vi "1D Scan.vi"(0 "System No.":i32=1 min=1 step=1, 1 "Analog In No.":i32=1 min=1 max=5 step=1, 2 "Axis to scan":string="Y", 4 "posdig":i16=4 caption="Digits" min=0 max=10 step=1, 5 "Scan direction":u16(ring) items=["Scan left & right (- & +)", "Scan only left (-)", "Scan only right (+)"], 6 "StartScan":bool, 7 "error in":errorcluster, 8 "Range":dbl=0.02 format="%.6f", 9 "Step size":dbl=0.002 format="%.6f", 12 "#6 polling?":bool=TRUE, 13 "Use MWG?":bool, 14 "VMO check?":bool=TRUE, 15 "Exit":bool, 16 "#5 Polling, ms":u32=10, 17 "Goto max":bool, 18 "Stop refnum":refnum<vi>) -> (20 "1D Array I":dbl[](array[numeric])=[0.00122, 0.00107, 0.00122, 0.00122, 0.56916, 1.88952, 3.75631, 5.80362, 5.80926, 3.7557, 1.89136, 0.56703, 0.00305, 0.00137, 0.00183] format="%.6f", 21 "1D Array X":dbl[](array[numeric])=[0.384, 0.386, 0.388, 0.39, 0.392, 0.394, 0.396, 0.398, 0.4, 0.402, 0.404, 0.406, 0.40800000000000003, 0.41000000000000003, 0.41200000000000003] format="%.6f", 23 "Intensity":cluster{dbl, dbl}(slide) scale=-1.0..0.00926 scale format="%.1f", 24 "Position":dbl format="%.6f", 27 "error out":errorcluster)   [LabVIEW 2011]
doc: "This VI performs a one-dimensional (1D) scan along one axis while monitoring an analog signal. The direction of the scan can be selected. After the scan, the axis to scan is optionally moved to the start position or to the position where the maximum occurred. The range and step size can be specified. After the scan, the axis can be moved to the maximum intensity position. Run XXX_Configuration_Setup.vi before starting this VI. \n\nStart the VI and select the system number (System No. = 1 in a one-system configuration) and Analog In number (Analog In No. = number of the analog channel to observe). Pressing Select will open a user interface which shows a list box with all axes connected to the selected system. Choose the axis to scan here or type the ID of the axis to scan directly into the Axis to scan control. Then, select Range and Step size for the scan. Digits is the number of digits after the decimal point in the position values that will be sent. #5 Polling is the cycle time in ms of the polling used to determine if motion has stopped after commanding a move. If this value is too large, scans may last very long. Set Scan orientation as needed (see possible orientations below). If #6 polling is on, VI will poll for position changes when idle. See control descriptions below to determine whether your system supports #6 polling. If MWG is on, the VI will use \"MWG.vi\" instead of \"MOV.vi\". This will result in a faster scan for systems which support the MWG command. See control descriptions below to determine if your system supports MWG. If VMO check is on, the VI will check whether the minimum and maximum position values of the scan line are within the system workspace before starting the scan. It is assumed that all positions between these points are reachable. See control descriptions below to determine whether your system supports VMO.\nIntensity graph shows the scanned intensity distribution. Autoscale can be switched on or off. If Autoscale is off, intensity is scaled from 0-10. \nPress Goto max to go to the position where the maximum intensity was found during the scan. With Clear max. the intensity value and the position value for the maximum intensity can be cleared. Press Save data to save scan data (axis, position and intensity information). Data will be saved in GCS Array format. With Save JPG a screen copy of this VI can be saved as a JPG file.\nPosition-Intensity Table will show the position value of the axis to scan and the corresponding intensity value which was captured during the scan. On the right side of the VI panel, the current and maximum intensity values and the current position value are shown.\nPress Stop to stop the scan and Exit to stop execution of this VI.\nTo use this VI as a sub-VI for your application without user interaction, wire the desired scan parameters (Axis to scan, Range, Step size, No. of pos. dig., #5 polling, #6 polling?, Use MWG?, VMO check?) to the corresponding terminals, and wire a TRUE constant to the Start scan, Goto max and Exit terminals. After calling the VI, it will make a scan, go to the maximum of the intensity distribution and finish execution. \n\nScan direction can be \n0: Left & right (- & +) meaning that the scan starts at \n(Start position - ½ Range) and stops at \n(Start position + ½ Range), \n1: To the left (-) meaning that scan starts at \n(Start position - Range) and stops at Start position, or \n2: To the right (+) meaning that scan starts at Start position and stops at (Start position + Range).\n\nWhen using as a sub-VI, connect Stop refnum terminal to stop VI from caller.\n\nValid for C-866, C-867, C-880, E-761, E-861, F-206, M-8X0, Mercury_GCS\n\nC-866: #6 polling? = FALSE, Use MWG? =FALSE, VMO check? =FALSE\nC-867: #6 polling? = FALSE, Use MWG? =FALSE, VMO check? =FALSE\nC-880: #6 polling? = TRUE, Use MWG? = FALSE, VMO check? = TRUE\nE-761: #6 polling? = TRUE, Use MWG? = FALSE, VMO check? = FALSE\nE-861: #6 polling? = FALSE, Use MWG? =FALSE, VMO check? =FALSE\nF-206: #6 polling? = TRUE, Use MWG? = TRUE, VMO check? = TRUE\nM-8X0: #6 polling? = TRUE, Use MWG? = FALSE, VMO check? = TRUE\nMercury_GCS: #6 polling? = FALSE, Use MWG? =FALSE, VMO check? = FALSE"
panel:
  in  "Save panel":bool
  in  "Autoscale":bool=TRUE
  out "No. of steps":i32=15
  out "Pos. Array":dbl[](array[numeric])=[0.398] caption="Start pos. array" format="%.6f"
  in  "Clear Max.":bool
  out "Start position":dbl=0.398 format="%.6f"
  out "Index of axis\nin Global 2":i32=1
  in  "Sub frame":i32=1
  in  "Select  axis":bool
  out "error":bool
  in  "StopAlign":bool
  in  "Next frame":i32
  in  "Save data":bool
  out "Position-Intensity Table":string[][](table)
  out "Intensity Graph":cluster{"1D Array X":dbl[], "1D Array Y":dbl[]}(graph) caption="No. of steps:"
  # "1D Scan"
  # "Run \"XXXX_Configuration_Setup.vi\" prior to running this VI. Scroll down for error clusters."
  # "Curr. I"
  # "Max. I"
  # "Error clusters and system specific settings"
  # "VI internal controls (do not change):"
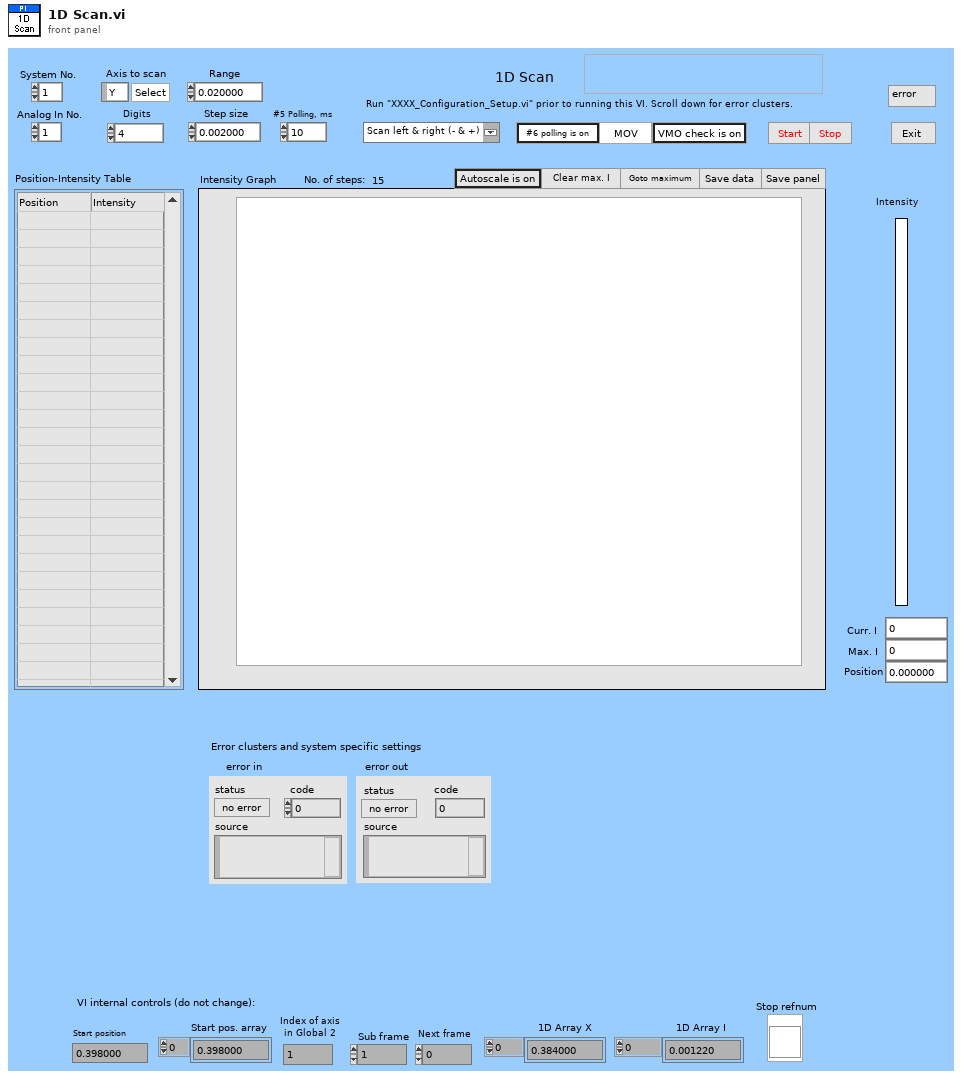
[diagram p1: front panel]
types:
  T1 = cluster{"Minimum":dbl, "Maximum":dbl, "Increment":dbl}
  T2 = cluster{"XName":string, "YName":string, "ZName":string}
  T3 = cluster{"Separator":string, "Remarks":string, "NDim":i32}
  T4 = cluster{"Read (F)/ Write":bool, "Path":path, "Datastream":string, "ArrayName":string}
  T5 = typedef "LVRectTypeDef.ctl" = cluster{"left":i16, "top":i16, "right":i16, "bottom":i16}
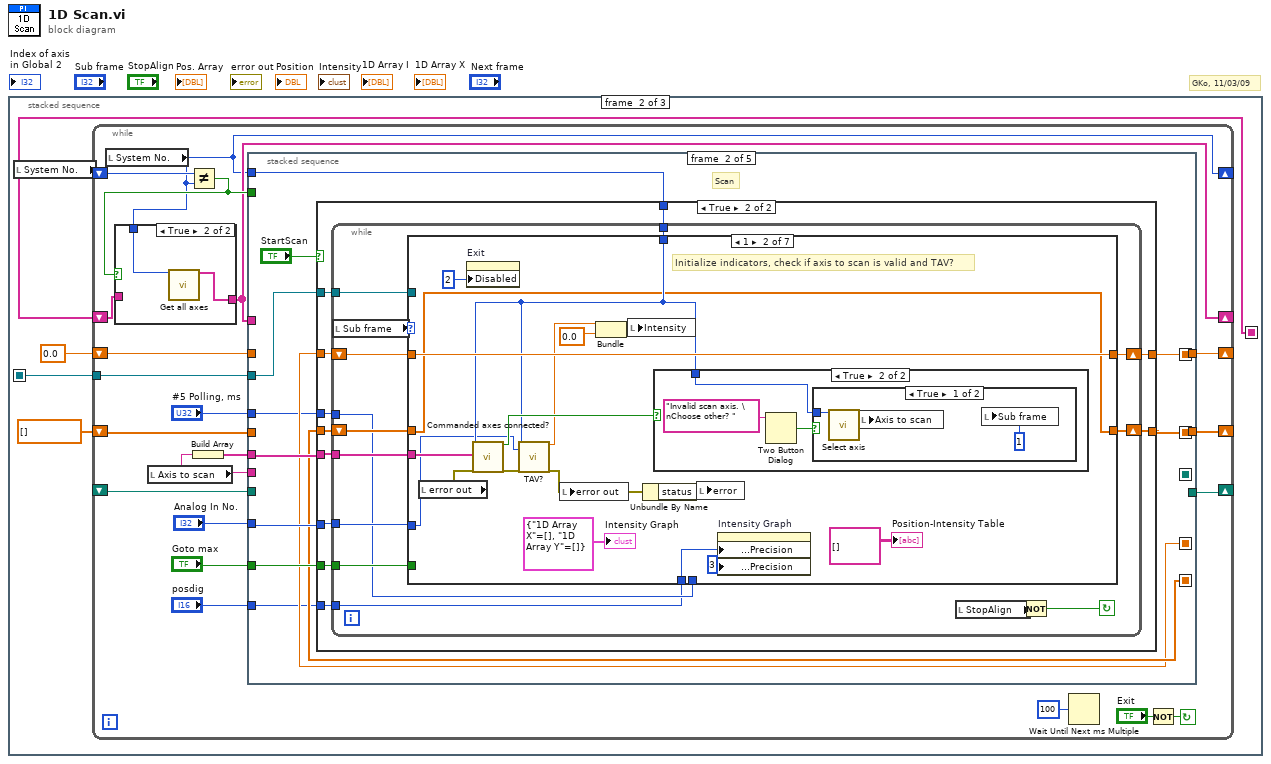
[diagram p0: block diagram]
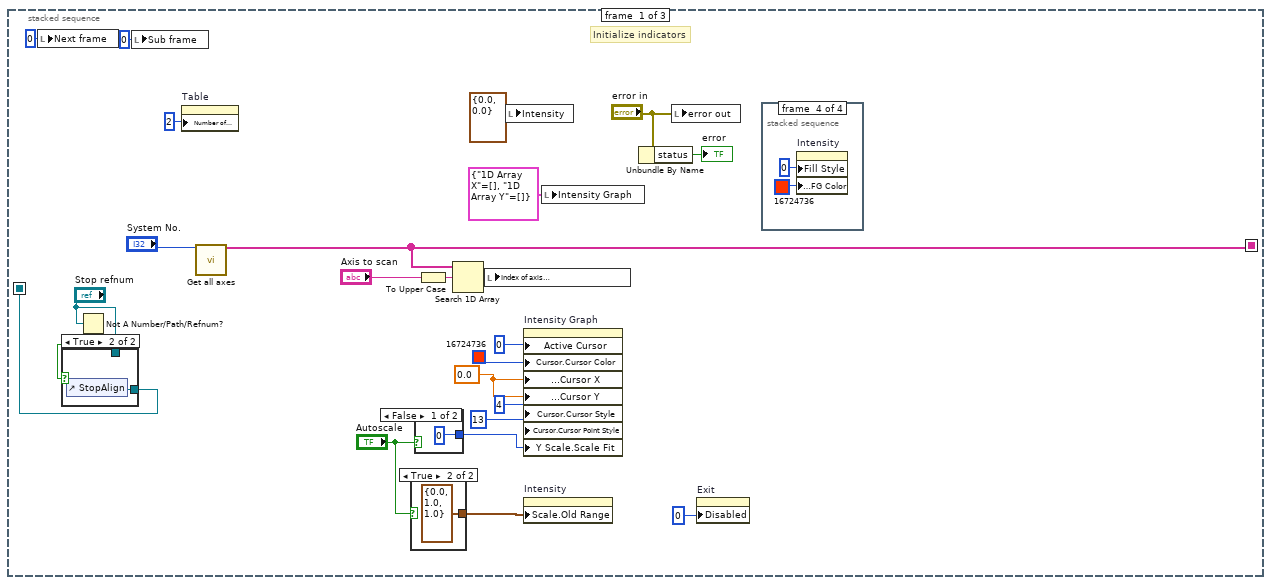
[diagram p2: hidden frame]
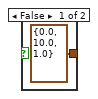
[diagram p3: hidden frame]
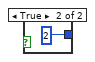
[diagram p5: hidden frame]
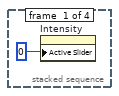
[diagram p6: hidden frame]
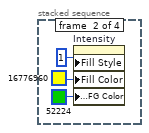
[diagram p7: hidden frame]
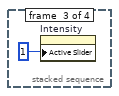
[diagram p8: hidden frame]
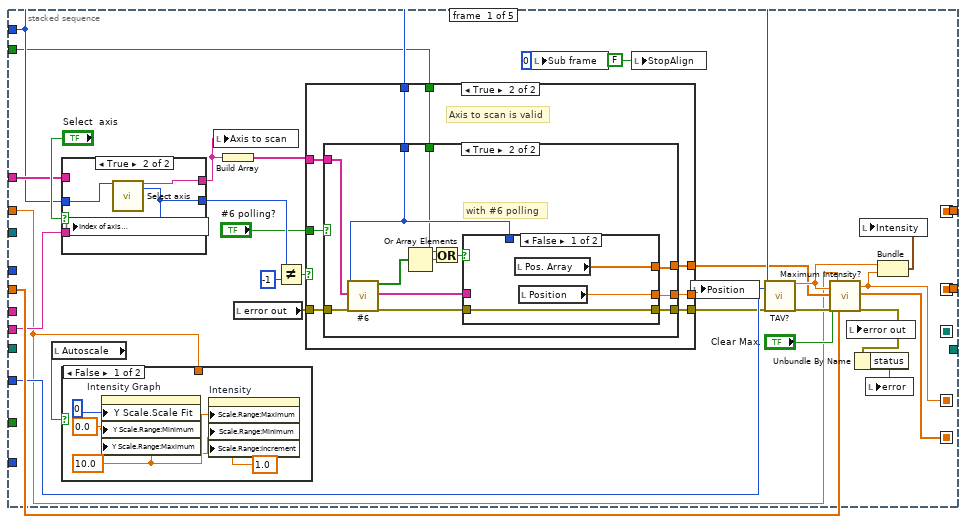
[diagram p9: hidden frame]
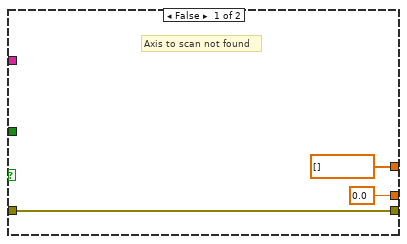
[diagram p10: hidden frame]
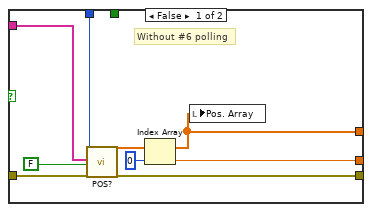
[diagram p11: hidden frame]
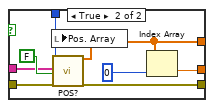
[diagram p12: hidden frame]
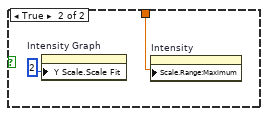
[diagram p13: hidden frame]
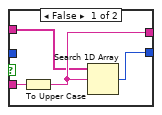
[diagram p14: hidden frame]
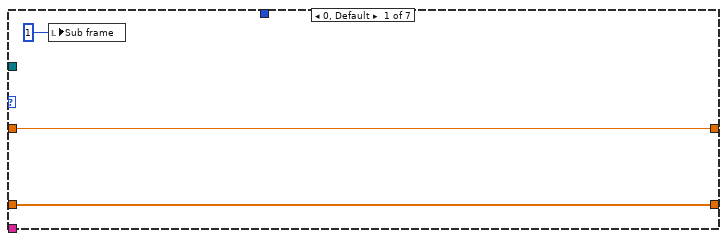
[diagram p16: hidden frame]
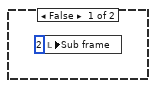
[diagram p17: hidden frame]
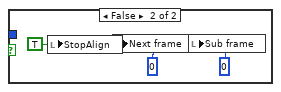
[diagram p18: hidden frame]
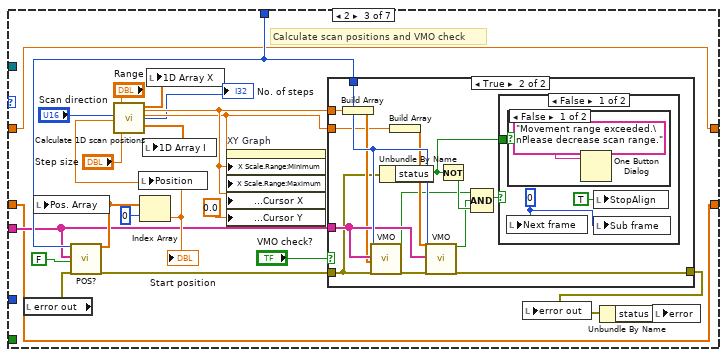
[diagram p19: hidden frame]
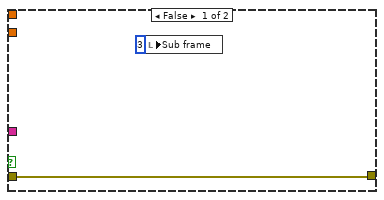
[diagram p20: hidden frame]
diagram:
  # "GKo, 11/03/09"
  n1 = stacked-sequence {
    seq-local: [w2 _ _] -> [_ w39 _]
    seq-local: [w5 _ _] -> [_ w38 _]
    frame #0 {
      w14 = 0.0 ("Write Attribute")
      # "Initialize indicators"
      n2 = local write "Next frame"(0 ("Next frame")) -> ()
      n3 = Not A Number/Path/Refnum?(number/path/refnum="Stop refnum") -> (NaN/Path/Refnum?=w7:bool)
      n4 = case shown="True" w7 {
        tunnel: [w27 w28] -> w5
        tunnel: "Stop refnum" -> [w27 _]
        frame False {
        }
        frame True {
          n5 = control-ref of="StopAlign"() -> (w28:refnum<vi>)
        }
      }
      n6 = local write "Sub frame"(0 ("Sub frame")) -> ()
      n7 = property on="Table" class="Tbl (strict)"("Number of Columns"=u32 2 ("Write Attribute")) -> ()  [unwired: 2 in, 2 out]
      n8 = call "Get all axes.vi"("System no."="System No.") -> ("Conn. Axes"=w2:string[])  [unwired: 18 in]
      n9 = case shown="True" "Autoscale" {
        tunnel: [T1 {"Minimum"=0.0, "Maximum"=10.0, "Increment"=1.0} ("Write Attribute") T1 {"Minimum"=0.0, "Maximum"=1.0, "Increment"=1.0} ("Write Attribute")] -> w21
        frame False {
        }
        frame True {
        }
      }
      n10 = case shown="False" "Autoscale" {
        tunnel: [u8 0 ("Write Attribute") u8 2 ("Write Attribute")] -> w10
        frame False {
        }
        frame True {
        }
      }
      n11 = To Upper Case(1:"Axis to scan") -> (0:w17:string)
      n12 = Search 1D Array(1D array=w2, element=w17) -> (index of element=w18:i32)  [unwired: 1 in]
      n13 = local write "Index of axis\nin Global 2"(w18) -> ()
      n14 = local write "Intensity"(cluster{dbl, dbl} {0.0, 0.0} ("Intensity")) -> ()
      n15 = property on="Intensity Graph" class="XYGraph (strict)"("Active Cursor"=u32 0 ("Write Attribute"), "Cursor.Cursor Color"=u32 16724736, "Cursor.Cursor Position:Cursor X"=w14, "Cursor.Cursor Position:Cursor Y"=w14, "Cursor.Cursor Style"=u8 4 ("Write Attribute"), "Cursor.Cursor Point Style"=u8 13 ("Write Attribute"), "Y Scale.Scale Fit"=w10) -> ()  [unwired: 2 in, 2 out]
      n16 = property on="Intensity" class="Slide (strict)"("Scale.Old Range"=w21) -> ()  [unwired: 2 in, 2 out]
      n17 = local write "Intensity Graph"(cluster{"1D Array X":dbl[], "1D Array Y":dbl[]} {"1D Array X"=[], "1D Array Y"=[]} ("Intensity Graph")) -> ()
      n18 = Unbundle By Name("error in") -> ("status"=→"error":bool)
      n19 = local write "error out"("error in") -> ()
      n20 = property on="Exit" class="Bool (strict)"("Disabled"=u8 0) -> ()  [unwired: 2 in, 2 out]
      n21 = stacked-sequence {
        frame #0 {
          n22 = property on="Intensity" class="Slide (strict)"("Active Slider"=0 ("Write Attribute")) -> ()  [unwired: 2 in, 2 out]
        }
        frame #1 {
          n23 = property on="Intensity" class="Slide (strict)"("Fill Style"=1 ("Write Attribute"), "Fill Color"=u32 16776960, "Slider Colors:FG Color"=u32 52224) -> ()  [unwired: 2 in, 2 out]
        }
        frame #2 {
          n24 = property on="Intensity" class="Slide (strict)"("Active Slider"=1 ("Write Attribute")) -> ()  [unwired: 2 in, 2 out]
        }
        frame #3 {
          n25 = property on="Intensity" class="Slide (strict)"("Fill Style"=0 ("Write Attribute"), "Slider Colors:FG Color"=u32 16724736) -> ()  [unwired: 2 in, 2 out]
        }
      }
    }
    frame #1 {
      n26 = local read "System No."() -> (w40:i32)
      n27 = while {
        tunnel: w38 -> [w44]
        shift-left: _ -> [w46]
        shift-right: [w45] -> _
        shift-left: w39 -> [w56]
        shift-right: [w55] -> _
        shift-left: w40 -> [w58]
        shift-right: [w43] -> _
        shift-left: dbl[] [] ("Position for I(max, out)") -> [w59]
        shift-right: [w51] -> _
        shift-left: 0.0 ("I(max, out)") -> [w60]
        shift-right: [w50] -> _
        stop <- w62 continue-if-true
        n28 = local read "System No."() -> (w43:i32)
        n29 = local read "Axis to scan"() -> (w52:string)
        n30 = Not Equal?(x=w58, y=w43) -> (x != y?=w57:bool)
        n31 = case shown="True" w57 {
          tunnel: [w474 w475] -> w55
          tunnel: w56 -> [w474 _]
          tunnel: w43 -> [_ w476]
          frame False {
          }
          frame True {
            n32 = call "Get all axes.vi"("System no."=w476) -> ("Conn. Axes"=w475:string[])  [unwired: 18 in]
          }
        }
        n33 = Build Array(w52) -> (w53:string[])
        n34 = stacked-sequence {
          seq-local: [w67 _ _ _ _] -> [_ w152 _ _ _]
          seq-local: [w78 _ _ _ _] -> [_ w153 _ _ _]
          seq-local: [_ w151 _ _ _] -> [_ _ w378 _ _]
          seq-local: [_ w150 _ _ _] -> [_ _ w379 _ _]
          seq-local: [_ _ _ w403 _] -> [_ _ _ _ w446]
          tunnel: w60 -> [w64 _ _ _ _]
          tunnel: w59 -> [w88 _ _ _ _]
          tunnel: w43 -> [w75 w157 w380 _ _]
          tunnel: w57 -> [w70 _ _ _ _]
          tunnel: w55 -> [w80 _ _ _ _]
          tunnel: "Goto max" -> [_ w156 w383 _ _]
          tunnel: w53 -> [_ w155 w382 _ _]
          tunnel: w52 -> [w77 _ _ w405 _]
          tunnel: "Analog In No." -> [w76 w154 w381 _ _]
          tunnel: [_ _ w379 _ _] -> w51
          tunnel: [_ _ w378 _ _] -> w50
          tunnel: "#5 Polling, ms" -> [_ w149 w377 _ _]
          tunnel: "posdig" -> [_ w148 w376 _ _]
          tunnel: w46 -> [_ _ _ w404 _]
          tunnel: [_ _ _ _ w445] -> w45
          tunnel: w44 -> [_ w147 w375 _ _]
          frame #0 {
            n35 = local read "Autoscale"() -> (w79:bool)
            n36 = case shown="True" "Select  axis" {
              tunnel: [w142 w146] -> w91
              tunnel: w75 -> [_ w145]
              tunnel: [w143 w144] -> w85
              tunnel: w80 -> [w141 _]
              tunnel: w77 -> [w140 _]
              frame False {
                n37 = To Upper Case(1:w140) -> (0:w142:string)
                n38 = Search 1D Array(1D array=w141, element=w142) -> (index of element=w143:i32)  [unwired: 1 in]
              }
              frame True {
                n39 = call "Select axis.vi"("System No."=w145) -> ("Selected axis"=w146:string, "Index of axis\nin Global 2"=w144:i32)  [unwired: 16 in, 1 out]
                n40 = local write "Index of axis\nin Global 2"(w144) -> ()
              }
            }
            n41 = case shown="False" w79 {
              tunnel: w64 -> [_ w138]
              frame False {
                w136 = 10.0 ("Write Attribute")
                w135 = 0.0 ("Write Attribute")
                n42 = property on="Intensity Graph" class="XYGraph (strict)"("Y Scale.Scale Fit"=u8 0 ("Write Attribute"), "Y Scale.Range:Minimum"=w135, "Y Scale.Range:Maximum"=w136) -> ()  [unwired: 2 in, 2 out]
                n43 = property on="Intensity" class="Slide (strict)"("Scale.Range:Maximum"=w136, "Scale.Range:Minimum"=w135, "Scale.Range:Increment"=1.0) -> ()  [unwired: 2 in, 2 out]
              }
              frame True {
                n44 = property on="Intensity Graph" class="XYGraph (strict)"("Y Scale.Scale Fit"=u8 2 ("Write Attribute")) -> ()  [unwired: 2 in, 2 out]
                n45 = property on="Intensity" class="Slide (strict)"("Scale.Range:Maximum"=w138) -> ()  [unwired: 2 in, 2 out]
              }
            }
            n46 = local write "Axis to scan"(w91) -> ()
            n47 = Build Array(w91) -> (w74:string[])
            n48 = local read "error out"() -> (w72:errorcluster)
            n49 = Not Equal?(x=w85, y=-1) -> (x != y?=w68:bool)
            n50 = case shown="True" w68 {
              tunnel: w74 -> [_ w103]
              tunnel: "#6 polling?" -> [_ w102]
              tunnel: w75 -> [_ w101]
              tunnel: w72 -> [w95 w100]
              tunnel: [w95 w99] -> w71
              tunnel: [dbl[] [] ("Position") w98] -> w66
              tunnel: [0.0 ("Numeric") w97] -> w69
              tunnel: w70 -> [_ w96]
              frame False {
                # "Axis to scan not found"
              }
              frame True {
                # "Axis to scan is valid"
                n51 = case shown="True" w102 {
                  tunnel: w101 -> [w109 w115]
                  tunnel: w103 -> [w108 w122]
                  tunnel: w100 -> [w107 w120]
                  tunnel: [w106 w119] -> w99
                  tunnel: [w105 w118] -> w98
                  tunnel: [w104 w116] -> w97
                  tunnel: w96 -> [_ w112]
                  frame False {
                    # "Without #6 polling"
                    n52 = call "POS?.vi"("System no."=w109, "Axes to query"=w108, "All axes?"=FALSE, "error in"=w107) -> ("Position"=w105:dbl[], "error out"=w106:errorcluster)  [unwired: 14 in]
                    n53 = Index Array(array=w105, index=0 ("Index")) -> (element=w104:dbl)
                    n54 = local write "Pos. Array"(w105) -> ()
                  }
                  frame True {
                    # "with #6 polling"
                    n55 = call "#6.vi"("System no."=w115, "error in"=w120) -> ("Pos change?"=w117:bool[], "error out"=w121:errorcluster)  [unwired: 16 in]
                    n56 = Or Array Elements(Boolean array=w117) -> (logical OR=w114:bool)
                    n57 = Or(x=w112, y=w114) -> (x .or. y?=w113:bool)
                    n58 = case shown="False" w113 {
                      tunnel: w122 -> [_ w131]
                      tunnel: w115 -> [_ w130]
                      tunnel: w121 -> [w125 w129]
                      tunnel: [w125 w128] -> w119
                      tunnel: [w124 w126] -> w118
                      tunnel: [w123 w127] -> w116
                      frame False {
                        n59 = local read "Pos. Array"() -> (w124:dbl[])
                        n60 = local read "Position"() -> (w123:dbl)
                      }
                      frame True {
                        n61 = call "POS?.vi"("System no."=w130, "Axes to query"=w131, "All axes?"=FALSE, "error in"=w129) -> ("Position"=w126:dbl[], "error out"=w128:errorcluster)  [unwired: 14 in]
                        n62 = local write "Pos. Array"(w126) -> ()
                        n63 = Index Array(array=w126, index=0 ("Index")) -> (element=w127:dbl)
                      }
                    }
                  }
                }
              }
            }
            n64 = local write "Sub frame"(0 ("Sub frame")) -> ()
            n65 = local write "StopAlign"(FALSE ("StopAlign")) -> ()
            n66 = local write "Position"(w69) -> ()
            n67 = call "TAV?.vi"("System no."=w75, "Board"=w76, "error in"=w71) -> ("Analog value"=w87:dbl, "error out"=w90:errorcluster)  [unwired: 13 in, 2 out]
            n68 = call "Maximum Intensity?.vi"("I(in)"=w87, "Position for I(in)"=w66, "Clear Maximum"="Clear Max.", "error in"=w90, "I(max, in)"=w64, "Position for I(max, in)"=w88) -> ("I(max, out)"=w67:dbl, "Position for I(max, out)"=w78:dbl[], "error out"=w83:errorcluster)  [unwired: 10 in, 1 out]
            n69 = local write "error out"(w83) -> ()
            n70 = Unbundle By Name(w83) -> ("status"=w82:bool)
            n71 = local write "error"(w82) -> ()
            n72 = Bundle("Analog value"=w87, "I(max, out)"=w67) -> (w86:cluster{"Analog value":dbl, "I(max, out)":dbl})  [unwired: 1 in]
            n73 = local write "Intensity"(w86) -> ()
          }
          frame #1 {
            # "Scan"
            n74 = case shown="True" "StartScan" {
              tunnel: w157 -> [_ w171]
              tunnel: w152 -> [w160 w170]
              tunnel: w153 -> [w159 w169]
              tunnel: [w160 w168] -> w151
              tunnel: [w159 w167] -> w150
              tunnel: w156 -> [_ w166]
              tunnel: w155 -> [_ w165]
              tunnel: w154 -> [_ w164]
              tunnel: w149 -> [_ w163]
              tunnel: w148 -> [_ w162]
              tunnel: w147 -> [_ w161]
              frame False {
              }
              frame True {
                n75 = while {
                  tunnel: w161 -> [w172]
                  tunnel: w162 -> [w173]
                  tunnel: w163 -> [w174]
                  tunnel: w164 -> [w176]
                  tunnel: w165 -> [w177]
                  tunnel: w166 -> [w178]
                  shift-left: w169 -> [w181]
                  shift-right: [w180] -> w167
                  shift-left: w170 -> [w182]
                  shift-right: [w179] -> w168
                  tunnel: w171 -> [w185]
                  stop <- w184 continue-if-true
                  n76 = local read "Sub frame"() -> (w183:i32)
                  n77 = case shown="1" w183 {
                    tunnel: w185 -> [_ w197 w234 w277 _ w368 _]
                    tunnel: w177 -> [_ w202 w222 w271 _ w367 _]
                    tunnel: w182 -> [w187 w201 w217 _ w340 w366 w372]
                    tunnel: w181 -> [w186 w190 w218 _ w339 w365 w371]
                    tunnel: [w186 w190 w218 w268 w339 w364 w371] -> w180
                    tunnel: [w187 w201 w217 w269 w340 w363 w372] -> w179
                    tunnel: w176 -> [_ w196 _ w270 _ w362 _]
                    tunnel: w178 -> [_ _ _ _ w337 _ _]
                    tunnel: w174 -> [_ _ _ w265 _ w354 _]
                    tunnel: w173 -> [_ w194 _ w263 w336 w353 _]
                    tunnel: w172 -> [_ _ _ w260 _ w352 _]
                    frame 0, Default {
                      n78 = local write "Sub frame"(1 ("Sub frame")) -> ()
                    }
                    frame 1 {
                      # "Initialize indicators, check if axis to scan is valid and TAV?"
                      n79 = local read "error out"() -> (w193:errorcluster)
                      n80 = property on="Exit" class="Bool (strict)"("Disabled"=u8 2) -> ()  [unwired: 2 in, 2 out]
                      n81 = call "Commanded axes connected?.vi"("System no."=w197, "Commanded axes"=w202, "error in"=w193) -> ("Controller error"=w204:bool, "error out"=w191:errorcluster)  [unwired: 15 in]
                      n82 = call "TAV?.vi"("System no."=w197, "Board"=w196, "error in"=w191) -> ("Analog value"=w199:dbl, "error out"=w192:errorcluster)  [unwired: 13 in, 2 out]
                      n83 = local write "error out"(w192) -> ()
                      n84 = Bundle("Analog value"=w199, "Analog value"=0.0) -> (w198:cluster{"Analog value":dbl, "Analog value":dbl})  [unwired: 1 in]
                      n85 = local write "Intensity"(w198) -> ()
                      n86 = Unbundle By Name(w192) -> ("status"=w203:bool)
                      n87 = case shown="True" w204 {
                        tunnel: w197 -> [_ w208]
                        frame False {
                          n88 = local write "Sub frame"(2 ("Sub frame")) -> ()
                        }
                        frame True {
                          n89 = Two Button Dialog(message="Invalid scan axis. \nChoose other? ") -> (T button?=w209:bool)  [unwired: 2 in]
                          n90 = case shown="True" w209 {
                            tunnel: w208 -> [w212 _]
                            frame True {
                              n91 = call "Select axis.vi"("System No."=w212) -> ("Selected axis"=w213:string)  [unwired: 16 in, 2 out]
                              n92 = local write "Axis to scan"(w213) -> ()
                              n93 = local write "Sub frame"(1 ("Sub frame")) -> ()
                            }
                            frame False {
                              n94 = local write "StopAlign"(TRUE ("StopAlign")) -> ()
                              n95 = local write "Next frame"(0 ("Next frame")) -> ()
                              n96 = local write "Sub frame"(0 ("Sub frame")) -> ()
                            }
                          }
                        }
                      }
                      n97 = local write "error"(w203) -> ()
                      n98 = property on="Intensity Graph" class="XYGraph (strict)"("X Scale.Display Format:Precision"=w194, "Y Scale.Display Format:Precision"=u8 3 ("Write Attribute")) -> ()  [unwired: 2 in, 2 out]
                      "Position-Intensity Table" <- string[][] [] ("Table")
                      "Intensity Graph" <- cluster{"1D Array X":dbl[], "1D Array Y":dbl[]} {"1D Array X"=[], "1D Array Y"=[]} ("XY Graph")
                    }
                    frame 2 {
                      # "Calculate scan positions and VMO check"
                      n99 = local read "error out"() -> (w237:errorcluster)
                      n100 = call "POS?.vi"("System no."=w234, "Axes to query"=w222, "All axes?"=FALSE, "error in"=w237) -> ("Position"=w223:dbl[], "error out"=w233:errorcluster)  [unwired: 14 in]
                      n101 = local write "Pos. Array"(w223) -> ()
                      n102 = Index Array(array=w223, index=0 ("Index")) -> (element=w231:dbl)
                      "Start position" <- w231
                      n103 = call "Calculate 1D scan positions.vi"("Scan direction"="Scan direction", "Start position"=w231, "Range"="Range", "Step size"="Step size") -> ("1D position array"=w230:dbl[], "Minimum position"=w228:dbl, "Maximum position"=w227:dbl, "No. of steps"=→"No. of steps":i32, "1D intensity array"=w229:dbl[])  [unwired: 11 in]
                      n104 = local write "Position"(w231) -> ()
                      n105 = local write "1D Array I"(w229) -> ()
                      n106 = local write "1D Array X"(w230) -> ()
                      n107 = property on="XY Graph" class="XYGraph (strict)"("X Scale.Range:Minimum"=w228, "X Scale.Range:Maximum"=w227, "Cursor.Cursor Position:Cursor X"=w228, "Cursor.Cursor Position:Cursor Y"=0.0 ("Write Attribute")) -> ()  [unwired: 2 in, 2 out]
                      n108 = case shown="True" "VMO check?" {
                        tunnel: w234 -> [_ w254]
                        tunnel: w222 -> [_ w253]
                        tunnel: w233 -> [w240 w245]
                        tunnel: w228 -> [_ w251]
                        tunnel: w227 -> [_ w249]
                        tunnel: [w240 w246] -> w225
                        frame False {
                          n109 = local write "Sub frame"(3 ("Sub frame")) -> ()
                        }
                        frame True {
                          n110 = Build Array(w251) -> (w250:dbl[])
                          n111 = call "VMO.vi"("System no."=w254, "Axes to command"=w253, "Position values"=w250, "error in"=w245) -> ("Move possible"=w243:bool, "error out"=w252:errorcluster)  [unwired: 14 in]
                          n112 = Unbundle By Name(w245) -> ("status"=w241:bool)
                          n113 = Build Array(w249) -> (w248:dbl[])
                          n114 = call "VMO.vi"("System no."=w254, "Axes to command"=w253, "Position values"=w248, "error in"=w252) -> ("Move possible"=w242:bool, "error out"=w246:errorcluster)  [unwired: 14 in]
                          n115 = Not(x=w241) -> (.not. x?=w244:bool)
                          n116 = Compound Arithmetic op=AND(w243, w242, w244) -> (w247:bool)
                          n117 = case shown="False" w247 {
                            tunnel: w241 -> [w255 _]
                            frame False {
                              w256 = 0 ("Next frame")
                              n118 = local write "Next frame"(w256) -> ()
                              n119 = case shown="False" w255 {
                                frame False {
                                n120 = One Button Dialog(message="Movement range exceeded.\nPlease decrease scan range.") -> ()  [unwired: 1 in, 1 out]
                                }
                                frame True {
                                }
                              }
                              n121 = local write "StopAlign"(TRUE ("StopAlign")) -> ()
                              n122 = local write "Sub frame"(w256) -> ()
                            }
                            frame True {
                              n123 = local write "Sub frame"(3 ("Sub frame")) -> ()
                            }
                          }
                        }
                      }
                      n124 = local write "error out"(w225) -> ()
                      n125 = Unbundle By Name(w225) -> ("status"=w224:bool)
                      n126 = local write "error"(w224) -> ()
                    }
                    frame 3 {
                      # "Scan"
                      n127 = local read "error out"() -> (w276:errorcluster)
                      n128 = local read "No. of steps"() -> (w266:i32)
                      n129 = local read "1D Array X"() -> (w278:dbl[])
                      n130 = local read "Pos. Array"() -> (w272:dbl[])
                      n131 = local read "1D Array I"() -> (w275:dbl[])
                      n132 = local write "Sub frame"(4 ("Sub frame")) -> ()
                      n133 = while {
                        tunnel: w260 -> [w279]
                        tunnel: w265 -> [w286]
                        tunnel: "Use MWG?" -> [w287]
                        tunnel: w266 -> [w288]
                        tunnel: w270 -> [w291]
                        tunnel: w271 -> [w292]
                        shift-left: w272 -> [w299]
                        shift-right: [w298] -> w268
                        shift-left: 0.0 ("I(max, out)") -> [w281]
                        shift-right: [w297] -> w269
                        shift-left: w275 -> [w304]
                        shift-right: [w293] -> w267
                        shift-left: w276 -> [w284]
                        shift-right: [w300] -> w262
                        tunnel: w263 -> [w303]
                        tunnel: w277 -> [w306]
                        tunnel: w278 -> [w294]
                        i -> [w285]
                        stop <- w310 continue-if-true
                        n134 = Index Array(array=w294, index=w285) -> (element=w289:dbl)
                        n135 = Increment(x=w285) -> (x+1=w308:i32)
                        n136 = Equal To 0?(x=w285) -> (x = 0?=w283:bool)
                        n137 = Less Or Equal?(x=w288, y=w308) -> (x <= y?=w307:bool)
                        n138 = local write "Position"(w289) -> ()
                        n139 = Build Array(w289) -> (w302:dbl[])
                        n140 = case shown="True" w283 {
                          tunnel: [u32 1 ("Wait befor TAV?, ms") u32 30 ("Wait befor TAV?, ms")] -> w282
                          frame False {
                          }
                          frame True {
                          }
                        }
                        n141 = case shown="False" w287 {
                          tunnel: w306 -> [w323 w334]
                          tunnel: w284 -> [w322 w333]
                          tunnel: w303 -> [w321 w332]
                          tunnel: w302 -> [w320 w331]
                          tunnel: [w319 w330] -> w301
                          tunnel: w292 -> [w318 w329]
                          tunnel: w291 -> [w317 w328]
                          tunnel: [w316 w327] -> w290
                          tunnel: w286 -> [w315 w326]
                          tunnel: w282 -> [w314 w325]
                          tunnel: w279 -> [w313 w324]
                          frame False {
                            n142 = call "MOV and TAV?.vi"("System no."=w323, "Board"=w317, "Axes to move"=w318, "Position values"=w320, "No.of digits"=w321, "error in"=w322, "Polling\nCycle time, ms"=w315, "Wait before\nTAV?, ms"=w314, "Stop refnum"=w313) -> ("Analog value"=w316:dbl, "error out"=w319:errorcluster)  [unwired: 9 in]
                          }
                          frame True {
                            n143 = call "MWG and TAV?.vi"("System no."=w334, "Board"=w328, "Axes to move"=w329, "Position values"=w331, "No.of digits"=w332, "error in"=w333, "Polling\nCycle time, ms"=w326, "Wait before\nTAV?, ms"=w325, "Stop refnum"=w324) -> ("Analog value"=w327:dbl, "error out"=w330:errorcluster)  [unwired: 9 in]
                          }
                        }
                        n144 = call "Maximum Intensity?.vi"("I(in)"=w290, "Position for I(in)"=w302, "error in"=w301, "I(max, in)"=w281, "Position for I(max, in)"=w299) -> ("I(max, out)"=w297:dbl, "Position for I(max, out)"=w298:dbl[], "error out"=w300:errorcluster)  [unwired: 11 in, 1 out]
                        n145 = Replace Array Subset(array=w304, new element=w290, index=w285) -> (w293:dbl[])
                        n146 = property class="Bool (strict)"(reference=w279) -> ("Value"=w280:bool)  [unwired: 1 in, 2 out]
                        n147 = property on="Intensity Graph" class="XYGraph (strict)"("Cursor.Cursor Position:Cursor X"=w289, "Cursor.Cursor Position:Cursor Y"=w290) -> ()  [unwired: 2 in, 2 out]
                        n148 = Bundle("Analog value"=w290, "I(max, out)"=w297) -> (w296:cluster{"Analog value":dbl, "I(max, out)":dbl})  [unwired: 1 in]
                        n149 = Bundle("1D Array X"=w294, "1D Array I"=w293) -> (w295:cluster{"1D Array X":dbl[], "1D Array I":dbl[]})  [unwired: 1 in]
                        n150 = Unbundle By Name(w300) -> ("status"=w305:bool)
                        n151 = local write "Intensity Graph"(w295) -> ()
                        n152 = Compound Arithmetic op=OR(w305, w307, w280) -> (w309:bool)
                        n153 = local write "Intensity"(w296) -> ()
                        n154 = Not(x=w309) -> (.not. x?=w310:bool)
                      }
                      n155 = local write "1D Array I"(w267) -> ()
                      n156 = local write "error out"(w262) -> ()
                      n157 = Unbundle By Name(w262) -> ("status"=w261:bool)
                      n158 = local write "error"(w261) -> ()
                    }
                    frame 4 {
                      w346 = FALSE ("use system decimal point (T)")
                      # "Update table"
                      n159 = case shown="True" w337 {
                        frame False {
                          n160 = local write "Sub frame"(5 ("Sub frame")) -> ()
                        }
                        frame True {
                          n161 = local write "Sub frame"(6 ("Sub frame")) -> ()
                        }
                      }
                      n162 = property on="Exit" class="Bool (strict)"("Disabled"=u8 0) -> ()  [unwired: 2 in, 2 out]
                      n163 = local read "1D Array X"() -> (w342:dbl[])
                      n164 = local read "1D Array I"() -> (w341:dbl[])
                      n165 = Number To Fractional String(use system decimal point (T)=w346, number=w341, precision (6)=i16 3) -> (F-format string=w345:string[])  [unwired: 1 in]
                      n166 = Number To Fractional String(use system decimal point (T)=w346, number=w342, precision (6)=w336) -> (F-format string=w347:string[])  [unwired: 1 in]
                      n167 = Build Array(w347, w345) -> (w344:string[][])
                      n168 = Transpose 2D Array(2D array=w344) -> (transposed array=w343:string[][])
                      n169 = local write "Position-Intensity Table"(w343) -> ()
                    }
                    frame 5 {
                      # "Return to start position"
                      n170 = local write "Sub frame"(6 ("Sub frame")) -> ()
                      n171 = local read "error out"() -> (w358:errorcluster)
                      n172 = local read "Pos. Array"() -> (w360:dbl[])
                      n173 = call "MOV and TAV?.vi"("System no."=w368, "Board"=w362, "Axes to move"=w367, "Position values"=w360, "No.of digits"=w353, "error in"=w358, "Polling\nCycle time, ms"=w354, "Wait before\nTAV?, ms"=u32 30 ("Wait befor TAV?, ms"), "Stop refnum"=w352) -> ("Analog value"=w350:dbl, "error out"=w361:errorcluster)  [unwired: 9 in]
                      n174 = local read "Start position"() -> (w351:dbl)
                      n175 = call "Maximum Intensity?.vi"("I(in)"=w350, "Position for I(in)"=w360, "error in"=w361, "I(max, in)"=w366, "Position for I(max, in)"=w365) -> ("I(max, out)"=w363:dbl, "Position for I(max, out)"=w364:dbl[], "error out"=w356:errorcluster)  [unwired: 11 in, 1 out]
                      n176 = local write "Position"(w351) -> ()
                      n177 = Bundle("Analog value"=w350, "I(max, out)"=w363) -> (w359:cluster{"Analog value":dbl, "I(max, out)":dbl})  [unwired: 1 in]
                      n178 = local write "Intensity"(w359) -> ()
                      n179 = local write "error out"(w356) -> ()
                      n180 = property on="Intensity Graph" class="XYGraph (strict)"("Cursor.Cursor Position:Cursor X"=w351, "Cursor.Cursor Position:Cursor Y"=w350) -> ()  [unwired: 2 in, 2 out]
                      n181 = Unbundle By Name(w356) -> ("status"=w357:bool)
                      n182 = local write "error"(w357) -> ()
                    }
                    frame 6 {
                      n183 = local write "Sub frame"(0 ("Sub frame")) -> ()
                      n184 = local write "Next frame"(0 ("Next frame")) -> ()
                      n185 = local write "StopAlign"(TRUE ("StopAlign")) -> ()
                    }
                  }
                  n186 = local read "StopAlign"() -> (w175:bool)
                  n187 = Not(x=w175) -> (.not. x?=w184:bool)
                }
              }
            }
          }
          frame #2 {
            # "Goto Maximum Intensity"
            n188 = case shown="False" w383 {
              tunnel: w379 -> [_ w395]
              tunnel: w382 -> [_ w393]
              tunnel: w381 -> [_ w392]
              tunnel: w380 -> [_ w391]
              tunnel: w378 -> [_ w390]
              tunnel: w377 -> [_ w389]
              tunnel: w376 -> [_ w387]
              tunnel: w375 -> [_ w386]
              frame False {
              }
              frame True {
                # "Goto max"
                n189 = local read "error out"() -> (w398:errorcluster)
                n190 = call "MOV and TAV?.vi"("System no."=w391, "Board"=w392, "Axes to move"=w393, "Position values"=w395, "No.of digits"=w387, "error in"=w398, "Polling\nCycle time, ms"=w389, "Wait before\nTAV?, ms"=u32 30 ("Wait befor TAV?, ms"), "Stop refnum"=w386) -> ("Analog value"=w384:dbl, "error out"=w400:errorcluster)  [unwired: 9 in]
                n191 = Index Array(array=w395, index=0 ("Index")) -> (element=w385:dbl)
                n192 = local write "Goto max"(FALSE ("Goto max")) -> ()
                n193 = local write "Position"(w385) -> ()
                n194 = call "Maximum Intensity?.vi"("I(in)"=w384, "Position for I(in)"=w395, "error in"=w400, "I(max, in)"=w390, "Position for I(max, in)"=w395) -> ("I(max, out)"=w399:dbl, "error out"=w397:errorcluster)  [unwired: 11 in, 2 out]
                n195 = local write "error out"(w397) -> ()
                n196 = property on="Intensity Graph" class="XYGraph (strict)"("Cursor.Cursor Position:Cursor X"=w385, "Cursor.Cursor Position:Cursor Y"=w384) -> ()  [unwired: 2 in, 2 out]
                n197 = Bundle("Analog value"=w384, "I(max, out)"=w399) -> (w401:cluster{"Analog value":dbl, "I(max, out)":dbl})  [unwired: 1 in]
                n198 = local write "Intensity"(w401) -> ()
                n199 = Unbundle By Name(w397) -> ("status"=w396:bool)
                n200 = local write "error"(w396) -> ()
              }
            }
          }
          frame #3 {
            n201 = case shown="True" "Save data" {
              tunnel: w405 -> [_ w413]
              tunnel: w404 -> [w407 w409]
              tunnel: [w407 w408] -> w403
              frame False {
              }
              frame True {
                # "Save data"
                n202 = call "File handler.vi"("Path in"=w409, "Read (F) or write (T)?"=TRUE ("New File?"), "Write new File?"=TRUE, "Extension"="txt", "With dialog?"=TRUE ("With dialog")) -> ("Path out"=w410:path, "Cancelled?"=w415:bool, "Data added?"=w414:bool)  [unwired: 12 in]
                n203 = case shown="False" w415 {
                  tunnel: w410 -> [w419 _]
                  tunnel: w414 -> [w433 _]
                  tunnel: w413 -> [w420 _]
                  tunnel: w409 -> [_ w444]
                  tunnel: [w419 w444] -> w408
                  frame False {
                    n204 = Get Date/Time String() -> (date string=w424:string, time string=w425:string)  [unwired: 3 in]
                    n205 = Concatenate Strings(w424, ", " ("Substring"), w425) -> (w421:string)
                    n206 = case shown="False" w433 {
                      tunnel: ["" ("ArrayName") w443] -> w432
                      tunnel: w421 -> [_ w443]
                      frame False {
                      }
                      frame True {
                      }
                    }
                    n207 = Bundle By Name(cluster=T4 {"Read (F)/ Write"=FALSE, "Path"=path "", "Datastream"="", "ArrayName"=""} ("IOSource"), "Read (F)/ Write"=TRUE, "Path"=w419, "ArrayName"=w432) -> (w439:T4)
                    n208 = Concatenate Strings("Generated by 1D Scan.vi, ", w421) -> (w422:string)
                    n209 = local read "1D Array X"() -> (w429:dbl[])
                    n210 = Bundle By Name(cluster=T3 {"Separator"="\t", "Remarks"="", "NDim"=0} ("Header in"), "Separator"="\t", "Remarks"=w422, "NDim"=2) -> (w436:T3)
                    n211 = local read "1D Array I"() -> (w428:dbl[])
                    n212 = Bundle By Name(cluster=T2 {"XName"="", "YName"="", "ZName"=""} ("Data names"), "XName"=w420, "YName"="Intensity") -> (w434:T2)
                    n213 = call "MatrixIO.vi"("IOSource"=w439, "XArray in"=w429, "YArray in"=w428, "Header in"=w436, "Data names"=w434) -> ("error out"=w431:errorcluster)  [unwired: 8 in, 6 out]
                    n214 = local write "error out"(w431) -> ()
                    n215 = Unbundle By Name(w431) -> ("status"=w430:bool)
                    n216 = local write "error"(w430) -> ()
                  }
                  frame True {
                  }
                }
              }
            }
          }
          frame #4 {
            n217 = case shown="False" "Save panel" {
              tunnel: w446 -> [w448 w449]
              tunnel: [w448 w450] -> w445
              frame False {
              }
              frame True {
                # "Save panel"
                n218 = call "File handler.vi"("Path in"=w449, "Read (F) or write (T)?"=TRUE ("New File?"), "Write new File?"=TRUE, "Extension"="jpg", "With dialog?"=TRUE ("Always with dialog")) -> ("Path out"=w451:path, "Cancelled?"=w454:bool)  [unwired: 12 in, 1 out]
                n219 = case shown="False" w454 {
                  tunnel: w451 -> [w457 _]
                  tunnel: [w457 w473] -> w450
                  tunnel: w449 -> [_ w473]
                  frame False {
                    w464 = 24 ("image depth")
                    n220 = local read "error in"() -> (w460:errorcluster)
                    n221 = Open VI Reference(vi path="1D Scan.vi", error in (no error)=w460) -> (vi reference=w470:refnum<vi>, error out=w471:errorcluster)  [unwired: 4 in]
                    n222 = invoke class="VI" method="FP.Old Get Image"(reference=w470, error in=w471, "visible area only"=TRUE, "image depth"=w464) -> (reference out=w472:refnum<vi>, error out=w463:errorcluster, "image"=w467:u8[], "colors"=w469:u32[], "bounds"=w468:T5)  [unwired: 4 in, 3 out]
                    n223 = call <vilib>:"Write JPEG File(6_1).vi"("quality (80)"=60, "color table"=w469, "depth"=w464, "error in (no error)"=w463, "flattened image data"=w467, "rect"=w468, "path to JPEG file"=w457) -> ("error out"=w462:errorcluster)  [unwired: 3 in, 1 out]
                    n224 = Close Reference(reference=w472, error in (no error)=w462) -> (error out=w459:errorcluster)
                    n225 = local write "error out"(w459) -> ()
                    n226 = Unbundle By Name(w459) -> ("status"=w458:bool)
                    n227 = local write "error"(w458) -> ()
                  }
                  frame True {
                  }
                }
              }
            }
          }
        }
        n228 = Wait Until Next ms Multiple(millisecond multiple=u32 100) -> ()  [unwired: 1 out]
        n229 = Not(x="Exit") -> (.not. x?=w62:bool)
      }
    }
    frame #2 {
      n230 = local write "Exit"(FALSE ("StopAlign")) -> ()
    }
  }
